vi "ClientSrv Set Client Title.vi"(7 "write access (none)":string) -> ()   [LabVIEW 2012]
doc: "This VI updates the title of the client window via VI server."
uses:
  glb_ClientSrv Globals.vi
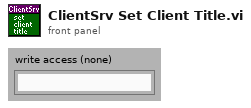
[diagram p1: front panel]
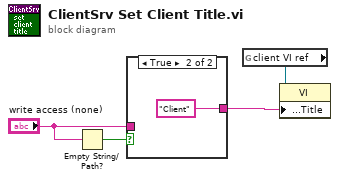
[diagram p0: block diagram]
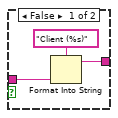
[diagram p2: hidden frame]
diagram:
  n1 = Empty String/Path?(string/path="write access (none)") -> (empty?=w4:bool)
  n2 = case shown="True" w4 {
    tunnel: "write access (none)" -> [w7 _]
    tunnel: [w5 "Client"] -> w2
    frame False {
      n3 = Format Into String(format string="Client (%s)", w7) -> (resulting string=w5:string)  [unwired: 2 in, 1 out]
    }
    frame True {
    }
  }
  n4 = global read "glb_ClientSrv Globals.vi" "client VI ref"() -> (w1:refnum<vi>)
  n5 = property class="VI"(reference=w1, "Front Panel Window:Title"=w2) -> ()  [unwired: 1 in, 2 out]
